vi "laba3.vi"() -> ()   [LabVIEW 2018]
panel:
  in  "количество элементов подмножества":i32
  in  "Старт подмножества":i32
  in  "Масштабный коэффициент":dbl
  out "Подмножества массива":dbl[](array[numeric])
  out "Конечный массив":dbl[](array[numeric])
  out "Массив случайных чисел":dbl[](array[numeric])
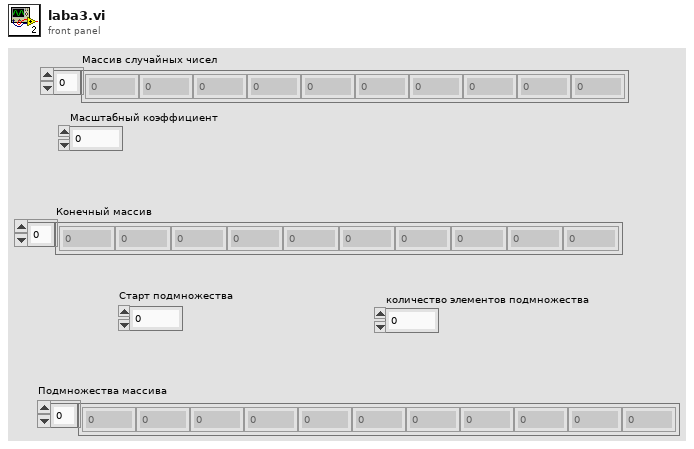
[diagram p1: front panel]
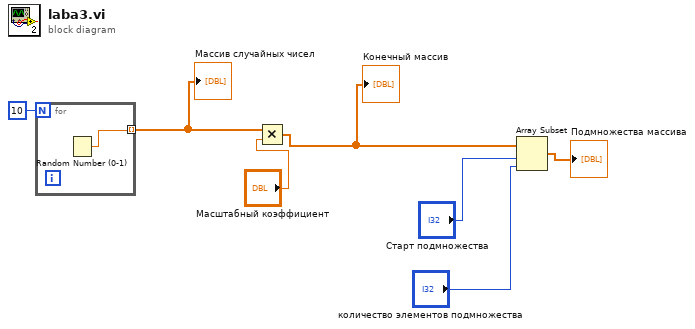
[diagram p0: block diagram]
diagram:
  n1 = for {
    N: 10 -> [_]
    tunnel: [w8] -> w6 mode=indexing
    n2 = Random Number (0-1)() -> (number: 0 to 1=w8:dbl)
  }
  "Массив случайных чисел" <- w6
  n3 = Multiply(x=w6, y="Масштабный коэффициент") -> (x*y=w4:dbl[])
  "Конечный массив" <- w4
  n4 = Array Subset(array=w4, index="Старт подмножества", length="количество элементов подмножества") -> (→"Подмножества массива":dbl[])
